vi "BackUpNetworkDisk.vi"(3 "Entrée d'erreur":errorcluster, 4 "ChaineInfoRefIn":refnum<vi>, 5 "NomProjet":string) -> (0 "error out":errorcluster, 1 "ChaineInfoRefOUT":refnum<vi>)   [LabVIEW 2017]
uses:
  DefDeType/WhichPath.ctl
panel:
  out "ProgressBar":i32(slide)
  # "BACK UP to Network DISK"
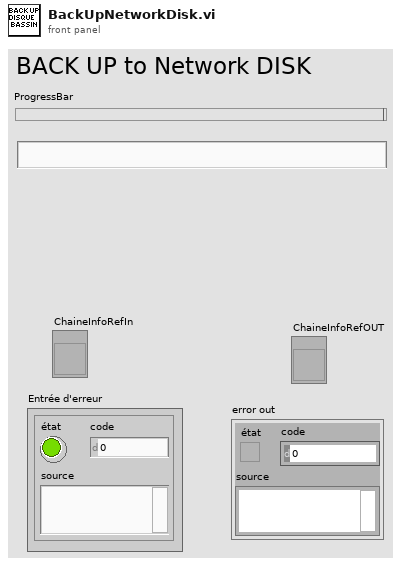
[diagram p1: front panel]
types:
  T1 = typedef "WhichPath.ctl" = enum16{"DossierProjet", "Config", "Meas", "MeasPCI", "MeasCRIO1", "MeasCRIO2", "MeasQualisys", "MeasHBM", "MeasTDMS", "Fig", "Res"}
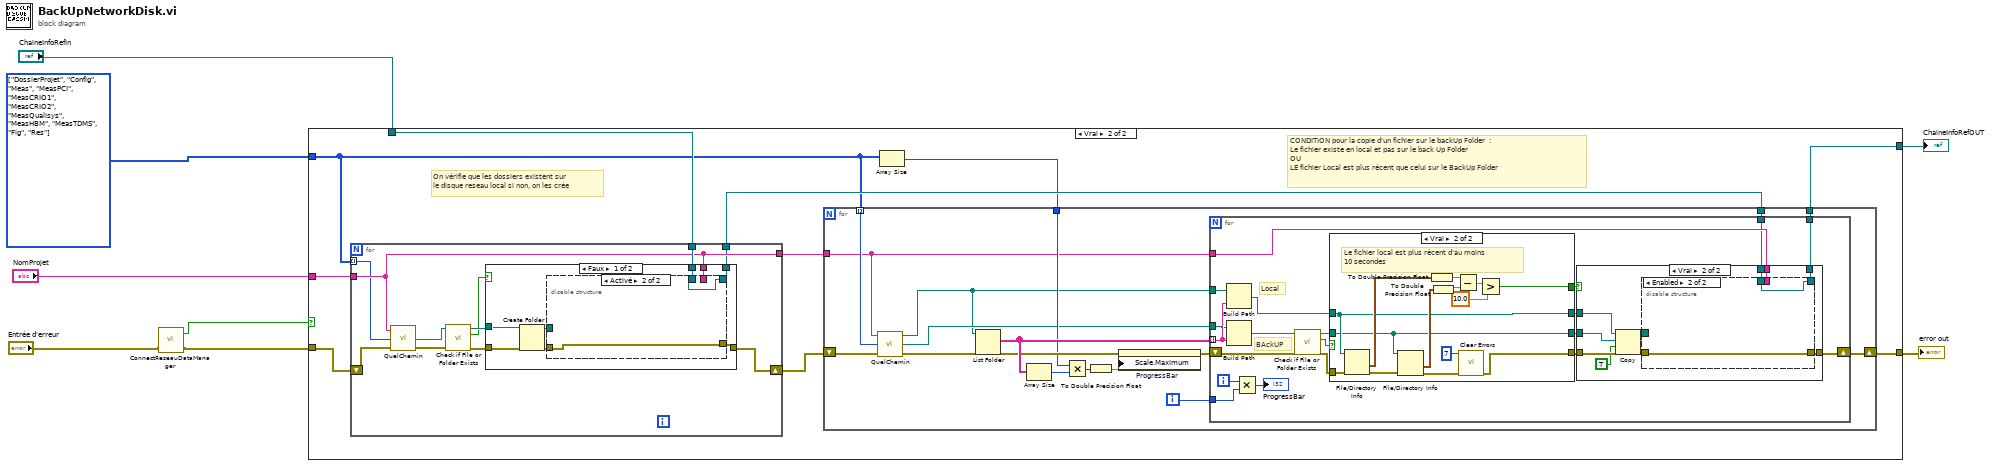
[diagram p0: block diagram]
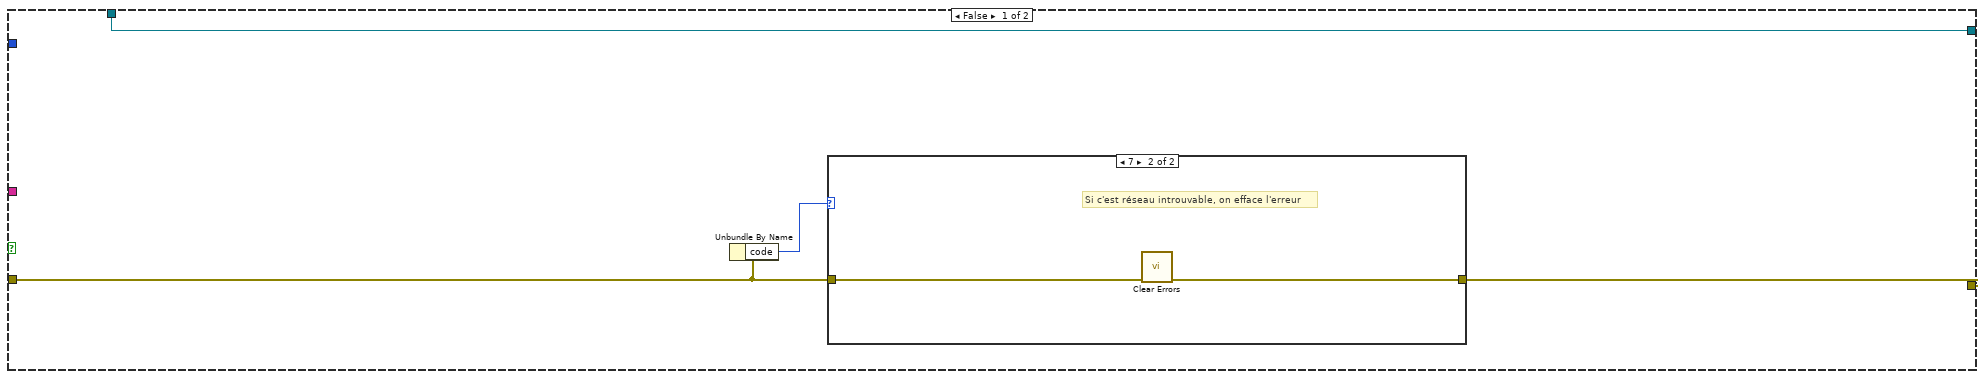
[diagram p2: hidden frame]
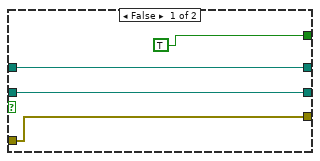
[diagram p4: hidden frame]
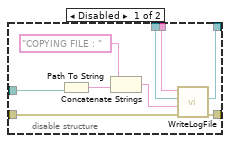
[diagram p6: hidden frame]
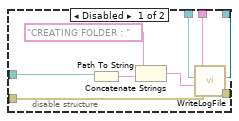
[diagram p7: hidden frame]
diagram:
  w1 = T1[] [enum."DossierProjet", enum."Config", enum."Meas", enum."MeasPCI", enum."MeasCRIO1", enum."MeasCRIO2", enum."MeasQualisys", enum."MeasHBM", enum."MeasTDMS", enum."Fig", enum."Res"] items=["DossierProjet", "Config", "Meas", "MeasPCI", "MeasCRIO1", "MeasCRIO2", "MeasQualisys", "MeasHBM", "MeasTDMS", "Fig", "Res"]
  n1 = call "ConnectReseauDataManager.vi"("entrée d'erreur"="Entrée d'erreur") -> ("sortie d'erreur"=w6:errorcluster, "Existe?"=w4:bool)  [unwired: 1 in]
  n2 = case shown="Vrai" w4 {
    tunnel: w6 -> [w11 w25]
    tunnel: [w12 w23] -> w8
    tunnel: "NomProjet" -> [_ w22]
    tunnel: w1 -> [_ w17]
    tunnel: "ChaineInfoRefIn" -> [w9 w19]
    tunnel: [w9 w20] -> w2
    frame False {
      n3 = Unbundle By Name(w11) -> ("code"=w10:i32)
      n4 = case shown="7" w10 {
        tunnel: [w13 w14] -> w12
        tunnel: w11 -> [w13 w15]
        frame 0, Default {
        }
        frame 7 {
          # "Si c'est réseau introuvable, on efface l'erreur"
          n5 = call <vilib>:"Clear Errors.vi"("error in (no error)"=w15) -> ("error out"=w14:errorcluster)  [unwired: 5 in, 1 out]
        }
      }
    }
    frame True {
      # "CONDITION pour la copie d'un fichier sur le backUp Folder  :\nLe fichier existe en local et pas sur le back Up Folder\nOU\nLE fichier Local est plus récent que celui sur le BackUp Folder"
      # "On vérifie que les dossiers existent sur \nle disque reseau local si non, on les crée"
      n6 = for {
        shift-right: [w110] -> w24
        shift-left: w25 -> [w111]
        tunnel: w22 -> [w107]
        tunnel: [w107] -> w21
        tunnel: w17 -> [w104] mode=indexing
        tunnel: w19 -> [w108]
        tunnel: [w106] -> w18
        n7 = call "QuelChemin.vi"("Entrée d'erreur"=w111, "WhichPath?"=w104, "NomProjet"=w107) -> ("Sortie d'erreur"=w109:errorcluster, "SurDisqueReseau"=w105:path)  [unwired: 1 out]
        n8 = call <vilib>:"Check if File or Folder Exists.vi"("error in (no error)"=w109, "path"=w105) -> ("error out"=w113:errorcluster, "file or folder exists?"=w112:bool, "dup path"=w114:path)  [unwired: 7 in]
        n9 = case shown="Faux" w112 {
          tunnel: w113 -> [w121 w135]
          tunnel: [w119 w135] -> w110
          tunnel: w114 -> [w122 _]
          tunnel: w108 -> [w118 w134]
          tunnel: w107 -> [w117 _]
          tunnel: [w115 w134] -> w106
          frame False {
            n10 = Create Folder(path (use dialog)=w122, error in=w121) -> (created path=w116:path, error out=w120:errorcluster)  [unwired: 1 in, 1 out]
            n11 = disable-structure shown="Activé" {
              disable-tunnel: w120 -> [w131 w133]
              disable-tunnel: [w130 w133] -> w119
              disable-tunnel: w118 -> [w129 w132]
              disable-tunnel: w117 -> [w128 _]
              disable-tunnel: w116 -> [w127 _]
              disable-tunnel: [w123 w132] -> w115
              frame Disabled {
                n12 = Path To String(path=w127) -> (string=w126:string)
                n13 = Concatenate Strings("CREATING FOLDER : " ("chaîne"), w126) -> (w125:string)
                n14 = call "WriteLogFile.vi"("entrée d'erreur"=w131, "Message"=w125, "ChaineInfoIN"=w129, "NomProjet"=w128) -> ("sortie d'erreur"=w130:errorcluster, "ChaineInfoOUT"=w123:refnum<vi>)  [unwired: 2 in]
              }
              frame Enabled {
              }
            }
          }
          frame True {
          }
        }
      }
      n15 = Array Size(array=w17) -> (size(s)=w16:i32)
      n16 = for {
        tunnel: w21 -> [w26]
        shift-right: [w41] -> w23
        shift-left: w24 -> [w42]
        tunnel: w17 -> [w40] mode=indexing
        tunnel: w18 -> [w39]
        tunnel: [w38] -> w20
        tunnel: w16 -> [w34]
        i -> [w30]
        n17 = call "QuelChemin.vi"("Entrée d'erreur"=w42, "WhichPath?"=w40, "NomProjet"=w26) -> ("Sortie d'erreur"=w27:errorcluster, "SurDisqueReseau"=w29:path, "SurDisqueLocal"=w28:path)
        n18 = List Folder(path=w28, error in=w27) -> (filenames=w37:string[], error out=w36:errorcluster)  [unwired: 2 in, 2 out]
        n19 = Array Size(array=w37) -> (size(s)=w33:i32)
        n20 = Multiply(x=w34, y=w33) -> (x*y=w32:i32)
        n21 = To Double Precision Float(number=w32) -> (double precision float=w31:dbl)
        n22 = property on="ProgressBar" class="Gliss (strict)"(error in=w36, "Scale.Maximum"=w31) -> (error out=w35:errorcluster)  [unwired: 1 in, 1 out]
        n23 = for {
          shift-right: [w58] -> w41
          shift-left: w35 -> [w62]
          tunnel: w37 -> [w59] mode=indexing
          tunnel: w28 -> [w60]
          tunnel: w29 -> [w57]
          tunnel: w26 -> [w48]
          tunnel: w39 -> [w47]
          tunnel: [w46] -> w38
          tunnel: w30 -> [w43]
          i -> [w45]
          # "BAckUP"
          # "Local"
          n24 = Build Path(base path=w60, name or relative path=w59) -> (appended path=w55:path)
          n25 = Build Path(base path=w57, name or relative path=w59) -> (appended path=w61:path)
          n26 = Multiply(x=w45, y=w43) -> (x*y=→"ProgressBar":i32)
          n27 = call <vilib>:"Check if File or Folder Exists.vi"("error in (no error)"=w62, "path"=w61) -> ("error out"=w56:errorcluster, "file or folder exists?"=w50:bool, "dup path"=w54:path)  [unwired: 7 in]
          n28 = case shown="Vrai" w50 {
            tunnel: w56 -> [w64 w80]
            tunnel: w55 -> [w66 w68]
            tunnel: w54 -> [w65 w67]
            tunnel: [w64 w77] -> w53
            tunnel: [w66 w68] -> w52
            tunnel: [w65 w67] -> w51
            tunnel: [TRUE w69] -> w49
            frame False {
            }
            frame True {
              # "Le fichier local est plus récent d'au moins \n10 secondes"
              n29 = File/Directory Info(path=w68, error in=w80) -> (last mod=w75:timestamp, error out=w79:errorcluster)  [unwired: 5 out]
              n30 = File/Directory Info(path=w67, error in=w79) -> (last mod=w74:timestamp, error out=w78:errorcluster)  [unwired: 5 out]
              n31 = To Double Precision Float(number=w75) -> (double precision float=w73:dbl)
              n32 = To Double Precision Float(number=w74) -> (double precision float=w72:dbl)
              n33 = Subtract(x=w73, y=w72) -> (x-y=w71:dbl)
              n34 = call <vilib>:"Clear Errors.vi"("error in (no error)"=w78, "specific error code to clear (0: all)"=7) -> ("error out"=w77:errorcluster)  [unwired: 4 in, 1 out]
              n35 = Greater?(x=w71, y=10.0) -> (0:w69:bool)
            }
          }
          n36 = case shown="Vrai" w49 {
            tunnel: w52 -> [_ w92]
            tunnel: w51 -> [_ w91]
            tunnel: [w82 w87] -> w58
            tunnel: w53 -> [w82 w90]
            tunnel: w48 -> [_ w86]
            tunnel: w47 -> [w81 w85]
            tunnel: [w81 w83] -> w46
            frame False {
            }
            frame True {
              n37 = Copy(8:w90, 9:TRUE ("écraser (F)"), 10:w91, 11:w92) -> (0:w88:errorcluster, 3:w84:path)  [unwired: 1 in, 1 out]
              n38 = disable-structure shown="Enabled" {
                disable-tunnel: w88 -> [w101 w103]
                disable-tunnel: [w100 w103] -> w87
                disable-tunnel: w86 -> [w99 _]
                disable-tunnel: w85 -> [w98 w102]
                disable-tunnel: w84 -> [w95 _]
                disable-tunnel: [w94 w102] -> w83
                frame Disabled {
                  n39 = Path To String(path=w95) -> (string=w97:string)
                  n40 = Concatenate Strings("COPYING FILE : " ("chaîne"), w97) -> (w93:string)
                  n41 = call "WriteLogFile.vi"("entrée d'erreur"=w101, "Message"=w93, "ChaineInfoIN"=w98, "NomProjet"=w99) -> ("sortie d'erreur"=w100:errorcluster, "ChaineInfoOUT"=w94:refnum<vi>)  [unwired: 2 in]
                }
                frame Enabled {
                }
              }
            }
          }
        }
      }
    }
  }
  "error out" <- w8
  "ChaineInfoRefOUT" <- w2
